vi "Motor Encoder Global.vi"() -> ()   [LabVIEW 2009]
panel:
  in  "Drive Speed Current (1-3.5)":fxp<+/-,18,8>
  in  "Drive Speed Control Feedback Gain":fxp<+/-,13,4>
  in  "Drive Speed Set Point (ft/sec)":fxp<+/-,18,8>
  in  "Drive Encoder Delta":i32
  in  "Steering Position Offset":i32
  in  "Steering Position Set Point (degrees)":i32
  in  "Steering Proportional Control Feedback Gain":fxp<+/-,20,5>
  in  "stop":bool
  out "Lidar Encoder Index":bool
  out "Steering Encoder Index":bool
  out "Drive Encoder Index":bool
  out "Lidar Encoder B":bool
  out "Steering Encoder B":bool
  out "Drive Encoder B":bool
  out "Lidar Encoder A":bool
  out "Steering Encoder A":bool
  out "Drive Encoder A":bool
  in  "Lidar Encoder":i32
  in  "Steering Encoder":i32
  in  "Drive Encoder":i32
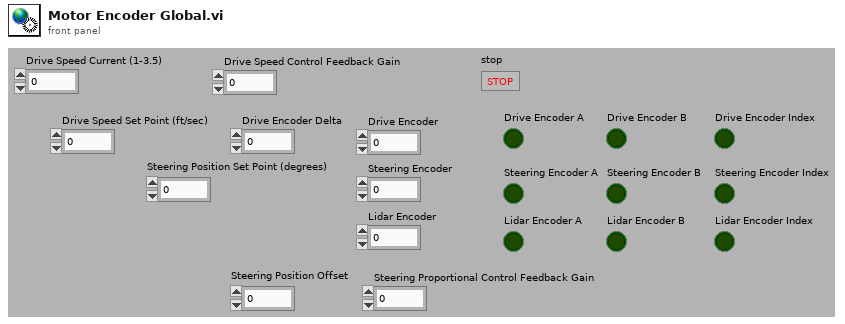
[diagram p1: front panel]
diagram:
